vi "noVIPM_IncrementBuild.vi"() -> ()   [LabVIEW 2019]
uses:
  <vilib>/Wiresmith Technology/G CLI/Argument Parser/Option Class/Option Configuration.ctl
  <vilib>/Wiresmith Technology/G CLI/Argument Parser/Option Class/Argument Type.ctl
  <vilib>/Wiresmith Technology/G CLI/CLI Class/CLI.lvclass
  <vilib>/Wiresmith Technology/G CLI/Argument Parser/Option Set Class/Option Set.lvclass
  <vilib>/Wiresmith Technology/G CLI/Argument Parser/Option Class/Option.lvclass
  VIPM/VIPM.lvlib
panel:
  out "error out":errorcluster
  out "VIPB File":path
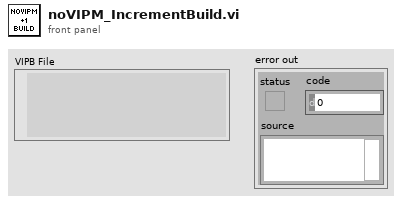
[diagram p1: front panel]
types:
  T1 = typedef "Option Parser.lvlib/Option.lvclass/Option Configuration.ctl" = cluster{"Option Type":T2, "Option Labels":string[], "Key":string, "Description":string, "Required":bool, "Default Value":string}
  T2 = typedef "Option Parser.lvlib/Option.lvclass/Argument Type.ctl" = enum16{"flag", "value"}
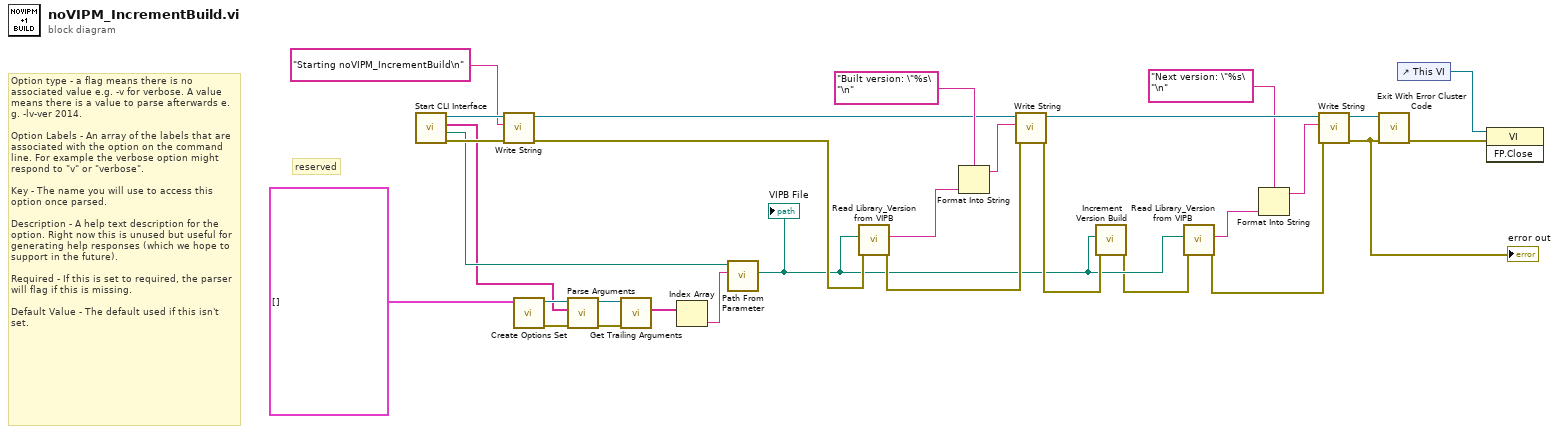
[diagram p0: block diagram]
diagram:
  # "Option type - a flag means there is no associated value e.g. -v for verbose. A value means there is a value to parse afterwards e.g. -lv-ver 2014.\n\nOption Labels - An array of the labels that are associated with the option on the command line. For example the verbose option might respond to \"v\" or \"verbose\".\n\nKey - The name you will use to access this option once parsed.\n\nDescription - A help text description for the option. Right now this is unused but useful for generating help responses (which we hope to support in the future).\n\nRequired - If this is set to required, the parser will flag if this is missing.\n\nDefault Value - The default used if this isn't set."
  # "reserved"
  n1 = call <vilib>:"Start CLI Interface.vi"() -> ("error out"=w28:errorcluster, "Working Directory"=w15:path, "Custom Parameters"=w4:string[], "CLI out"=w30:refnum<class "CLI.lvclass">)  [unwired: 8 in]
  n2 = call <vilib>:"Write String.vi"("error in (no error)"=w28, "Text to Write"="Starting noVIPM_IncrementBuild\n" ("format string"), "CLI in"=w30) -> ("error out"=w10:errorcluster, "CLI out"=w24:refnum<class "CLI.lvclass">)  [unwired: 7 in]
  n3 = call <vilib>:"Create Options Set.vi"("Options"=T1[] []) -> ("error out"=w20:errorcluster, "Option Set out"=w18:refnum<class "Option Set.lvclass">)  [unwired: 9 in]
  n4 = call <vilib>:"Parse Arguments.vi"("error in (no error)"=w20, "Arguments"=w4, "Option Set in"=w18) -> ("error out"=w19:errorcluster, "Option Set out"=w16:refnum<class "Option Set.lvclass">)  [unwired: 5 in, 2 out]
  n5 = call <vilib>:"Get Trailing Arguments.vi"("error in (no error)"=w19, "Option Set in"=w16) -> ("Arguments"=w17:string[])  [unwired: 7 in, 2 out]
  n6 = Index Array(array=w17) -> (element=w27:string)  [unwired: 1 in]
  n7 = call <vilib>:"Path From Parameter.vi"("Path Parameter"=w27, "Working Directory"=w15) -> ("Full Path"=w3:path)  [unwired: 9 in]
  "VIPB File" <- w3
  n8 = call "Read Library_Version from VIPB.vi"("error in"=w10, "VIPB File Path"=w3) -> ("error out"=w9:errorcluster, "Library_Version"=w13:string)  [unwired: 8 in]
  n9 = Format Into String(format string="Built version: \"%s\"\n", w13) -> (resulting string=w23:string)  [unwired: 2 in, 1 out]
  n10 = call <vilib>:"Write String.vi"("error in (no error)"=w9, "Text to Write"=w23, "CLI in"=w24) -> ("error out"=w8:errorcluster, "CLI out"=w22:refnum<class "CLI.lvclass">)  [unwired: 7 in]
  n11 = call "Increment Version Build.vi"("error in (no error)"=w8, "path"=w3) -> ("error out"=w2:errorcluster)  [unwired: 9 in]
  n12 = call "Read Library_Version from VIPB.vi"("error in"=w2, "VIPB File Path"=w3) -> ("error out"=w7:errorcluster, "Library_Version"=w11:string)  [unwired: 8 in]
  n13 = Format Into String(format string="Next version: \"%s\"\n", w11) -> (resulting string=w6:string)  [unwired: 2 in, 1 out]
  n14 = call <vilib>:"Write String.vi"("error in (no error)"=w7, "Text to Write"=w6, "CLI in"=w22) -> ("error out"=w1:errorcluster, "CLI out"=w26:refnum<class "CLI.lvclass">)  [unwired: 7 in]
  "error out" <- w1
  n15 = call <vilib>:"Exit With Error Cluster Code.vi"("error in (no error)"=w1, "CLI in"=w26) -> ("error out"=w21:errorcluster)  [unwired: 9 in]
  n16 = control-ref of="This VI"() -> (w5:refnum<vi>)
  n17 = invoke class="VI" method="FP.Close"(reference=w5, error in=w21) -> ()  [unwired: 1 in, 3 out]
